vi "Introduction Demo_Global_Init.vi"(11 "Object":T1) -> ()   [LabVIEW 2015]
uses:
  <resource>/Framework/Providers/API/ItemRef.ctl
  <resource>/Framework/Providers/API/mxLvMenuItem.ctl
panel:
  out "error out":errorcluster
  in  "error in":errorcluster
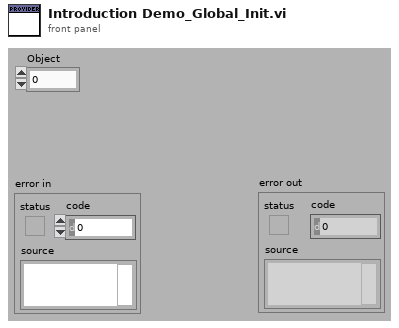
[diagram p1: front panel]
types:
  T1 = typedef "ItemRef.ctl" = u64
  T2 = typedef "mxLvMenuItem.ctl" = cluster{"Menu Name":string, "Description":string, "Icon File Name":path, "Menu Tag":string, "Enabled":bool, "Checked":bool, "Separator":bool, "Batchable":bool, "Weight":i32, "Batch Mode (Ignored if Not Batchable)":enum32{"Show If All Items Support Command", "Show If Any Items Support Command"}, "Menu Location":enum32{"<None>", "Project", "Project / Build Specifications", "Tools", "Tools / Source Control", "Tools / Real-Time Module", "Help"}, "Exclude From Getting Started Window Menu":bool}
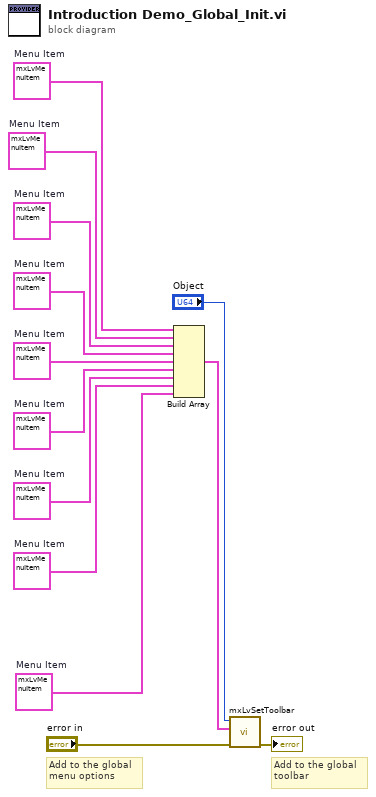
[diagram p0: block diagram]
diagram:
  w1 = T2 {"Menu Name"="GDevCon/Toolbar/Our Giants are Female", "Description"="Our Giants are Female", "Icon File Name"=path "../Icons/GDevCon Logo png.png", "Menu Tag"="Our Giants are Female", "Enabled"=TRUE, "Checked"=FALSE, "Separator"=TRUE, "Batchable"=TRUE, "Weight"=0, "Batch Mode (Ignored if Not Batchable)"=enum."Show If All Items Support Command", "Menu Location"=enum."<None>", "Exclude From Getting Started Window Menu"=TRUE}  # Menu Item
  w2 = T2 {"Menu Name"="GDevCon/Toolbar/Menu Items", "Description"="Menu Items2", "Icon File Name"=path "../Icons/GDevCon Logo png.png", "Menu Tag"="Menu Items2", "Enabled"=TRUE, "Checked"=FALSE, "Separator"=FALSE, "Batchable"=TRUE, "Weight"=0, "Batch Mode (Ignored if Not Batchable)"=enum."Show If All Items Support Command", "Menu Location"=enum."<None>", "Exclude From Getting Started Window Menu"=TRUE}  # Menu Item
  w3 = T2 {"Menu Name"="GDevCon/Toolbar/Quick Drop Shortcut", "Description"="Quick Drop Shortcut2", "Icon File Name"=path "../Icons/GDevCon Logo png.png", "Menu Tag"="Quick Drop Shortcut2", "Enabled"=TRUE, "Checked"=FALSE, "Separator"=FALSE, "Batchable"=TRUE, "Weight"=0, "Batch Mode (Ignored if Not Batchable)"=enum."Show If All Items Support Command", "Menu Location"=enum."<None>", "Exclude From Getting Started Window Menu"=TRUE}  # Menu Item
  w4 = T2 {"Menu Name"="GDevCon/Toolbar/Right Click Menu", "Description"="Right Click Menu2", "Icon File Name"=path "../Icons/GDevCon Logo png.png", "Menu Tag"="Right Click Menu2", "Enabled"=TRUE, "Checked"=FALSE, "Separator"=FALSE, "Batchable"=TRUE, "Weight"=0, "Batch Mode (Ignored if Not Batchable)"=enum."Show If All Items Support Command", "Menu Location"=enum."<None>", "Exclude From Getting Started Window Menu"=TRUE}  # Menu Item
  w5 = T2 {"Menu Name"="GDevCon/Toolbar/Introduction Demos/Menu Items", "Description"="Menu Items", "Icon File Name"=path "../Icons/GDevCon Logo png.png", "Menu Tag"="Menu Items", "Enabled"=TRUE, "Checked"=FALSE, "Separator"=FALSE, "Batchable"=TRUE, "Weight"=0, "Batch Mode (Ignored if Not Batchable)"=enum."Show If All Items Support Command", "Menu Location"=enum."<None>", "Exclude From Getting Started Window Menu"=TRUE}  # Menu Item
  w6 = T2 {"Menu Name"="GDevCon/Toolbar/Introduction Demos/Quick Drop Shortcut", "Description"="Quick Drop Shortcut", "Icon File Name"=path "../Icons/GDevCon Logo png.png", "Menu Tag"="Quick Drop Shortcut", "Enabled"=TRUE, "Checked"=FALSE, "Separator"=FALSE, "Batchable"=TRUE, "Weight"=0, "Batch Mode (Ignored if Not Batchable)"=enum."Show If All Items Support Command", "Menu Location"=enum."<None>", "Exclude From Getting Started Window Menu"=TRUE}  # Menu Item
  w7 = T2 {"Menu Name"="GDevCon/Toolbar/Introduction Demos/Right Click Menu", "Description"="Right Click Menu", "Icon File Name"=path "../Icons/GDevCon Logo png.png", "Menu Tag"="Right Click Menu", "Enabled"=TRUE, "Checked"=FALSE, "Separator"=FALSE, "Batchable"=TRUE, "Weight"=0, "Batch Mode (Ignored if Not Batchable)"=enum."Show If All Items Support Command", "Menu Location"=enum."<None>", "Exclude From Getting Started Window Menu"=TRUE}  # Menu Item
  w8 = T2 {"Menu Name"="GDevCon/Toolbar/Introduction Demos/Icon Scripting", "Description"="Icon Scripting", "Icon File Name"=path "../Icons/GDevCon Logo png.png", "Menu Tag"="Icon Scripting", "Enabled"=TRUE, "Checked"=FALSE, "Separator"=FALSE, "Batchable"=TRUE, "Weight"=0, "Batch Mode (Ignored if Not Batchable)"=enum."Show If All Items Support Command", "Menu Location"=enum."<None>", "Exclude From Getting Started Window Menu"=TRUE}  # Menu Item
  w11 = T2 {"Menu Name"="GDevCon/Toolbar/Introduction Demos/Project Provider", "Description"="Project Provider", "Icon File Name"=path "../Icons/GDevCon Logo png.png", "Menu Tag"="Project Provider", "Enabled"=TRUE, "Checked"=TRUE, "Separator"=FALSE, "Batchable"=TRUE, "Weight"=0, "Batch Mode (Ignored if Not Batchable)"=enum."Show If All Items Support Command", "Menu Location"=enum."<None>", "Exclude From Getting Started Window Menu"=TRUE}  # Menu Item
  # "Add to the global\ntoolbar"
  # "Add to the global\nmenu options"
  n1 = Build Array(w11, w8, w7, w6, w5, w4, w3, w2, w1) -> (w13:T2[])
  n2 = call <resource>:"mxLvSetToolbar.vi"("error in"="error in", "Toolbar Items"=w13, "Item"="Object") -> ("error out"=→"error out":errorcluster)  [unwired: 7 in, 1 out]
